vi "FTP.Disconnect.vi"(8 "error in (no error)":errorcluster, 11 "FTP Session out":T1) -> (0 "error out":errorcluster)   [LabVIEW 2016]
uses:
  <vilib>/FTP/ftp0.llb/FTP Session.ctl
  <vilib>/FTP/NI_FTP.lvlib
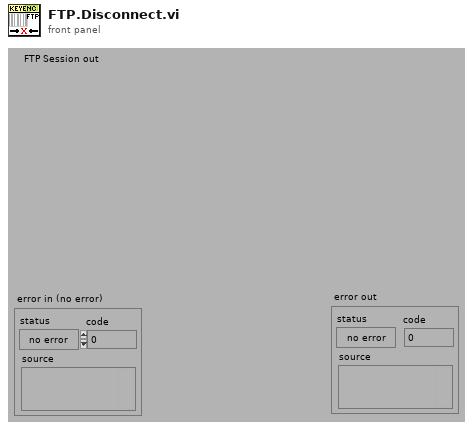
[diagram p1: front panel]
types:
  T1 = typedef "NI_FTP.lvlib/FTP Session.ctl" = refnum<k5>
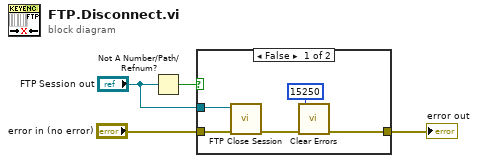
[diagram p0: block diagram]
diagram:
  n1 = Not A Number/Path/Refnum?(number/path/refnum="FTP Session out") -> (NaN/Path/Refnum?=w4:bool)
  n2 = case shown="False" w4 {
    tunnel: "FTP Session out" -> [w9 _]
    tunnel: [w5 w10] -> w1
    tunnel: "error in (no error)" -> [w8 w10]
    frame False {
      n3 = call <vilib>:"FTP Close Session.vi"("error in (no error)"=w8, "ftp session"=w9) -> ("error out"=w6:errorcluster)  [unwired: 6 in, 3 out]
      n4 = call <vilib>:"Clear Errors.vi"("error in (no error)"=w6, "specific error code to clear (0: all)"=15250) -> ("error out"=w5:errorcluster)  [unwired: 4 in, 1 out]
    }
    frame True {
    }
  }
  "error out" <- w1
